vi "Untitled 1.vi"(7 "error in (no error)":errorcluster) -> (21 "A/DI0 (N Samples) (Pin 11)":bool[](array[boolean]), 27 "error out":errorcluster)   [LabVIEW 2014]
doc: "Reads values from one or more digital input channels on the NI myRIO. Use this Express VI to read one or multiple samples for each channel at one time.\n--------------------\n\nThis Express VI is configured as follows:\n\nNode name: Digital input (n samples)\nChannel: A/DI0 (N Samples) (Pin 11) ; Custom Name: <blank>\nSample rate: 2,00\nSample Rate Unit: MHz\nSamples: 10000"
uses:
  <vilib>/myRIO/Common/Instrument Driver Framework/myRIO v1.0/DI Block/vis/myRIO v1.0 DI Block Read.vi
  <vilib>/Utility/error.llb/Error Cluster From Error Code.vi
  <vilib>/myRIO/Instrument Drivers/Onboard IO/DI Block/DI Block.lvlib
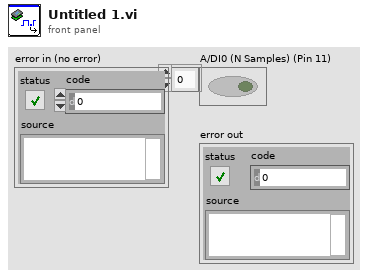
[diagram p1: front panel]
types:
  T1 = typedef "DI Block.lvlib/DI Block Reference.ctl" = cluster{"myRIO Reference":T2, "DI (N Samples) Channels List":T6}
  T2 = typedef "myRIO Generic Hardware Reference.ctl" = cluster{"myRIO Model":T3, "myRIO Hardware Reference":T4}
  T3 = typedef "Hardware Version Enum.ctl" = enum16{"Unknown", "myRIO-1900", "myRIO-1950"}
  T4 = typedef "myRIO v1.0 Reference.ctl" = cluster{"Generic FPGA Reference":T5, "Allow multiple opens":bool}
  T5 = typedef "Generic FPGA Reference.ctl" = refnum<k20>
  T6 = typedef "DI Block Channels List.ctl" = T7[]
  T7 = typedef "DI Block Channels Enum.ctl" = enum16{"Not Connected", "A/DI0 (N Samples)"}
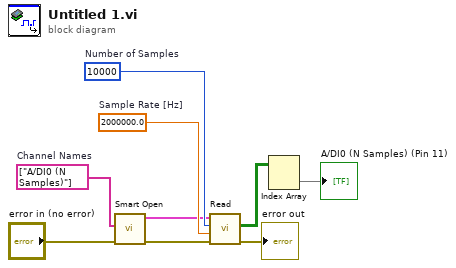
[diagram p0: block diagram]
diagram:
  w7 = 2000000.0  # Sample Rate [Hz]
  w8 = u32 10000  # Number of Samples
  w9 = tag[] ["A/DI0 (N Samples)"]  # Channel Names
  n1 = call <vilib>:"Smart Open.vi"("error in (no error)"="error in (no error)", "Channel Names"=w9) -> ("error out"=w2:errorcluster, "DI (N Samples) Ref Out"=w3:T1)  [unwired: 8 in]
  n2 = call <vilib>:"Read.vi"("error in (no error)"=w2, "Sample Rate [Hz]"=w7, "Number of Samples"=w8, "DI (N Samples) Ref In"=w3) -> ("error out"=→"error out":errorcluster, "Values"=w6:bool[][])  [unwired: 5 in, 1 out]
  n3 = Index Array(array=w6) -> (element=→"A/DI0 (N Samples) (Pin 11)":bool[])  [unwired: 2 in]
